vi "rethinkdb_handshake_initial.vi"(8 "error in (no error)":errorcluster, 10 "password":string, 11 "user":string) -> (0 "error out":errorcluster, 1 "client_first_message":string, 2 "dup password":string, 3 "initial_message":string)   [LabVIEW 2017]
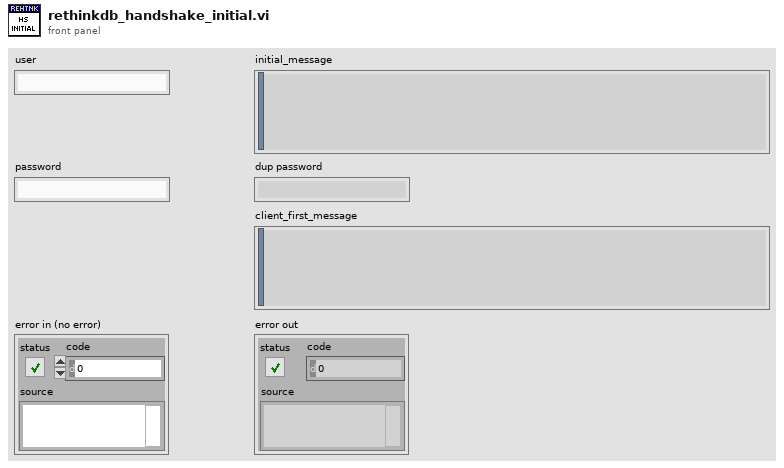
[diagram p1: front panel]
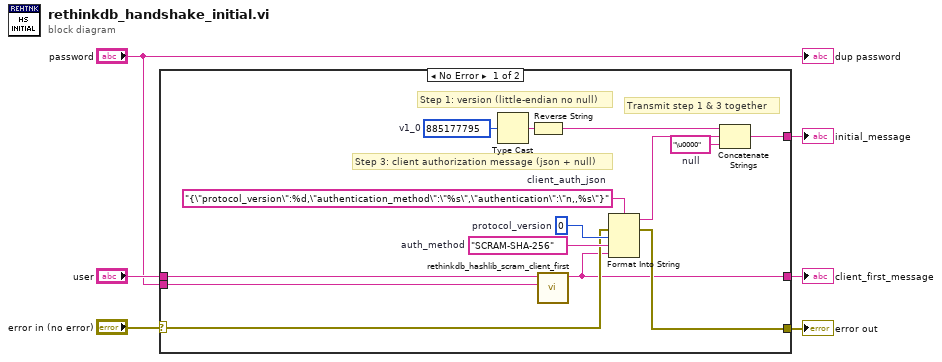
[diagram p0: block diagram]
diagram:
  n1 = case shown="No Error" "error in (no error)" {
    selector: "error in (no error)" -> [w10 w21]
    tunnel: "password" -> [w7 _]
    tunnel: "user" -> [w8 _]
    tunnel: [w12 w21] -> w4
    tunnel: [w18 _] -> w3
    tunnel: [w9 _] -> w2
    frame No Error {
      w13 = "SCRAM-SHA-256"  # auth_method
      w14 = 0  # protocol_version
      w15 = "{\"protocol_version\":%d,\"authentication_method\":\"%s\",\"authentication\":\"n,,%s\"}"  # client_auth_json
      w16 = "\u0000"  # null
      w20 = u32 885177795  # v1_0
      # "Step 3: client authorization message (json + null)"
      # "Transmit step 1 & 3 together"
      # "Step 1: version (little-endian no null)"
      n2 = Type Cast(x=w20) -> (*(type *) &x=w19:string)  [unwired: 1 in]
      n3 = Reverse String(1:w19) -> (0:w17:string)
      n4 = call "rethinkdb_hashlib_scram_client_first.vi"("password"=w7, "user"=w8) -> ("client_first_message"=w9:string)  [unwired: 9 in]
      n5 = Format Into String(format string=w15, error in=w10, w14, w13, w9) -> (resulting string=w11:string, error out=w12:errorcluster)  [unwired: 1 in]
      n6 = Concatenate Strings(w17, w11, w16) -> (w18:string)
    }
    frame Error {
    }
  }
  "error out" <- w4
  "initial_message" <- w3
  "client_first_message" <- w2
  "dup password" <- "password"
